vi "KH Control.vi"(8 "error in":errorcluster, 11 "KH7008":refnum<class "Instrument.KH7008.lvclass">) -> (0 "error out":errorcluster, 3 "KH7008.lvclass out":refnum<class "Instrument.KH7008.lvclass">)   [LabVIEW 2019, in "Instrument.KH7008.lvclass"]
uses:
  Instrument.KH7008.lvclass
  typedefs/SetAll-Array.ctl
  typedefs/SetAll-Cluster.ctl
  typedefs/Channel-Enum.ctl
  typedefs/Gain-Enum.ctl
  typedefs/Filter-Enum.ctl
  typedefs/Shunt-Enum.ctl
  typedefs/Coupling-Enum.ctl
  typedefs/Input Configuration-Enum.ctl
  C:/Program Files (x86)/National Instruments/LabVIEW 2019/user.lib/LevyLab/Levylab Instruments/SMOs/Instrument/Instrument.lvclass
  Instrument.KH7008.lvclass/Instrument.KH7008.ctl
  <userlib>/LevyLab/Levylab Instruments/SMOs/Instrument/Instrument.lvclass/Instrument.ctl
  <vilib>/MakerHub/Toolbox/LMH-Toolbox.lvlib
  C:/Program Files (x86)/National Instruments/LabVIEW 2019/vi.lib/JKI/JKI SMO/SMO/SMO.lvclass
  <userlib>/LevyLab/Levylab Instruments/SMOs/Instrument/Instrument.lvclass
panel:
  in  "OK":bool
  in  "Radio Buttons":T1(radio)
  in  "Address":string(combo)="COM3"
  in  "Channel Settings":T2
  # "Measure Current: Current, Shunt Resistor: 50kOhm\nMeasure Voltage: Voltage, Shunt Resistor: Open\nApplying Gate: Current, Shunt Resistor: 50kOhm\n                      Open all the unused gate\n\n1. Create a copy of drivers under C:\\Krohn-Hite 7008\\Drivers if there is none. \n2. In device manager browse the driver for Krohn-Hite \n\nWarning: repeated channels will cause false reading in the lock-in"
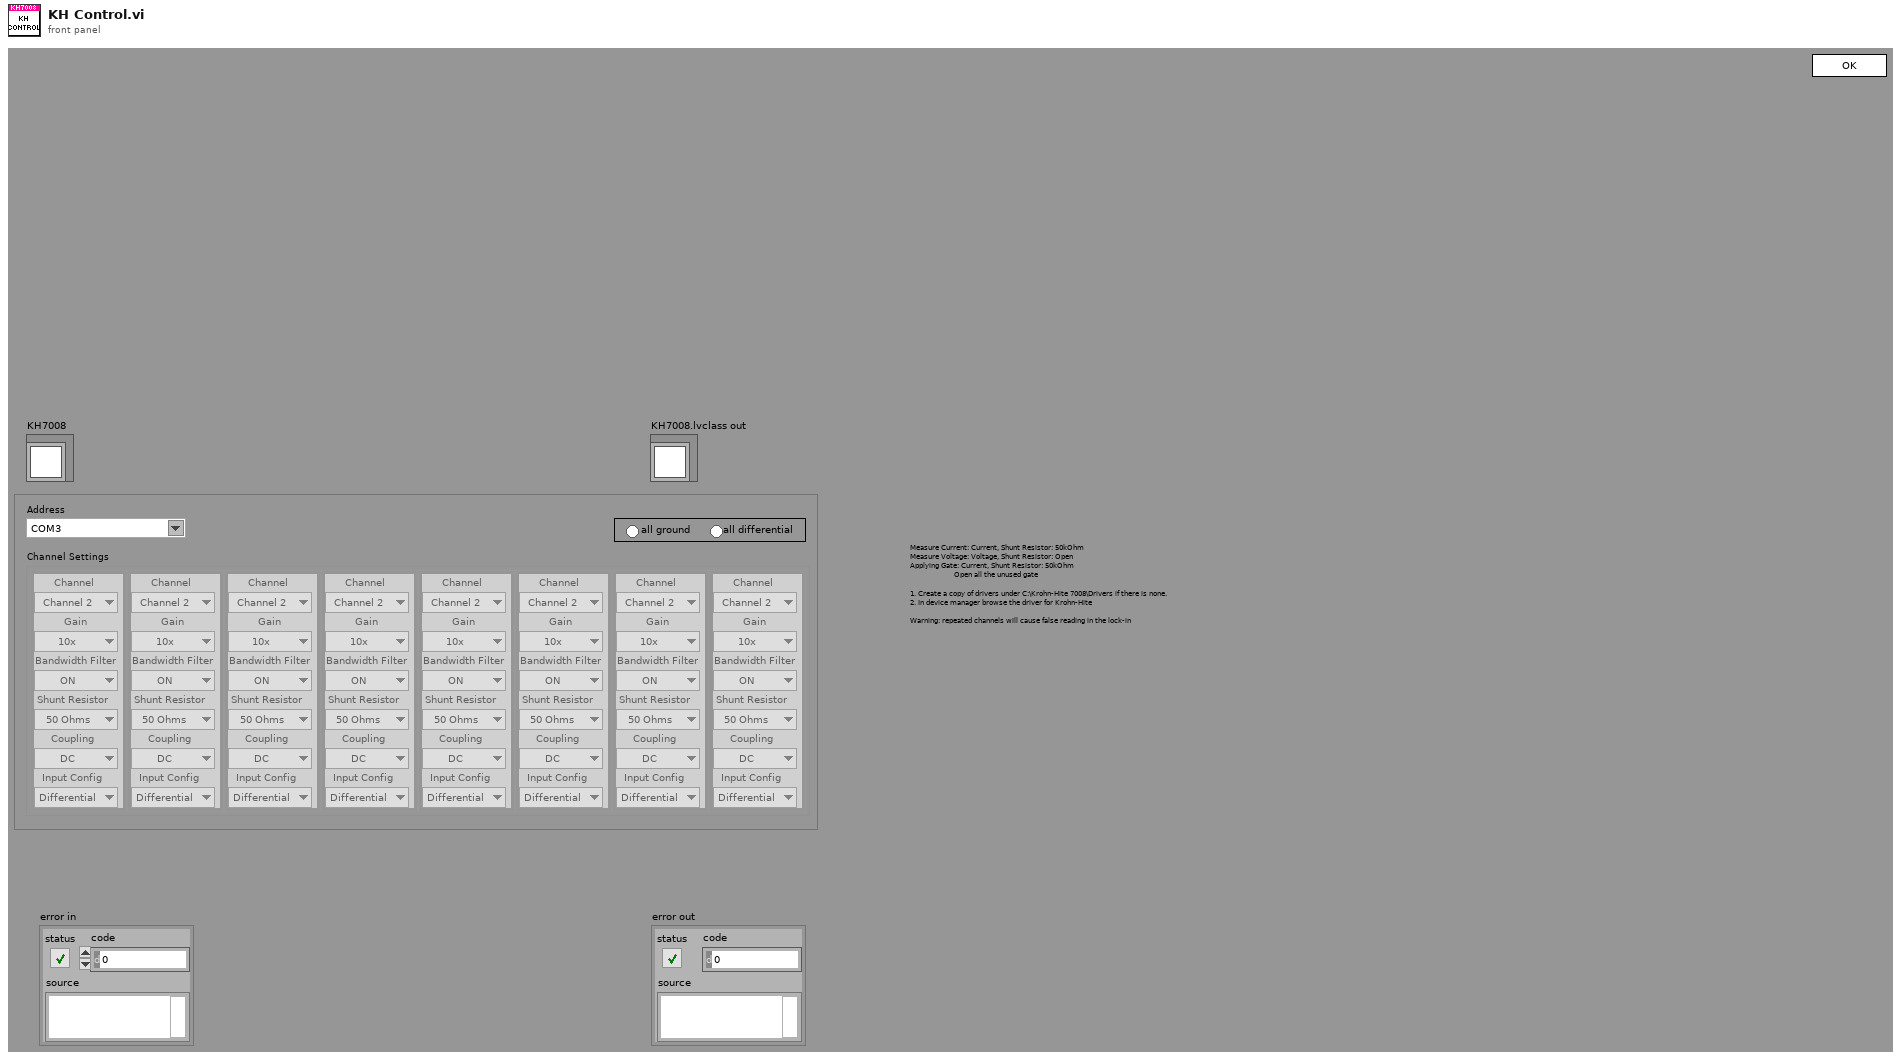
[diagram p1: front panel]
types:
  T1 = enum32{"No Selection", "all ground", "all differential"}
  T2 = typedef "Instrument.KH7008.lvclass/SetAll-Array.ctl" = T3[]
  T3 = typedef "Instrument.KH7008.lvclass/SetAll-Cluster.ctl" = cluster{"Channel":T4, "Gain":T5, "Bandwidth Filter":T6, "Shunt Resistor":T7, "Coupling":T8, "Input Config":T9}
  T4 = typedef "Instrument.KH7008.lvclass/Channel-Enum.ctl" = enum16{"Channel 1", "Channel 2", "Channel 3", "Channel 4", "Channel 5", "Channel 6", "Channel 7", "Channel 8"}
  T5 = typedef "Instrument.KH7008.lvclass/Gain-Enum.ctl" = enum16{"1x", "10x", "100x", "1000x"}
  T6 = typedef "Instrument.KH7008.lvclass/Filter-Enum.ctl" = enum16{"OFF", "ON"}
  T7 = typedef "Instrument.KH7008.lvclass/Shunt-Enum.ctl" = enum16{"Open", "50 Ohms", "500 Ohms", "5k Ohms", "50k Ohms", "10M Ohm"}
  T8 = typedef "Instrument.KH7008.lvclass/Coupling-Enum.ctl" = enum16{"AC", "DC"}
  T9 = typedef "Instrument.KH7008.lvclass/Input Configuration-Enum.ctl" = enum16{"Ground", "SE+ (-gnd)", "SE- (+gnd)", "Differential"}
  T10 = enum32{"Invalid", "Standard", "Closed", "Hidden", "Minimized", "Maximized"}
  T11 = enum32{"invalid app kind", "Development System", "Run Time System", "Student Edition", "Embedded LabVIEW", "Evaluation", "Custom"}
  T12 = cluster{"Core":cluster{"Current VI Reference":refnum<vi>, "Close Panel on Exit?":bool}, "KH7008":refnum<class "Instrument.KH7008.lvclass">, "Address":string, "Channel Setting":T3[]}
  T13 = cluster{"Current VI Reference":refnum<vi>, "Close Panel on Exit?":bool}
  T14 = enum32{"Bad", "Idle", "Run top level", "Running"}
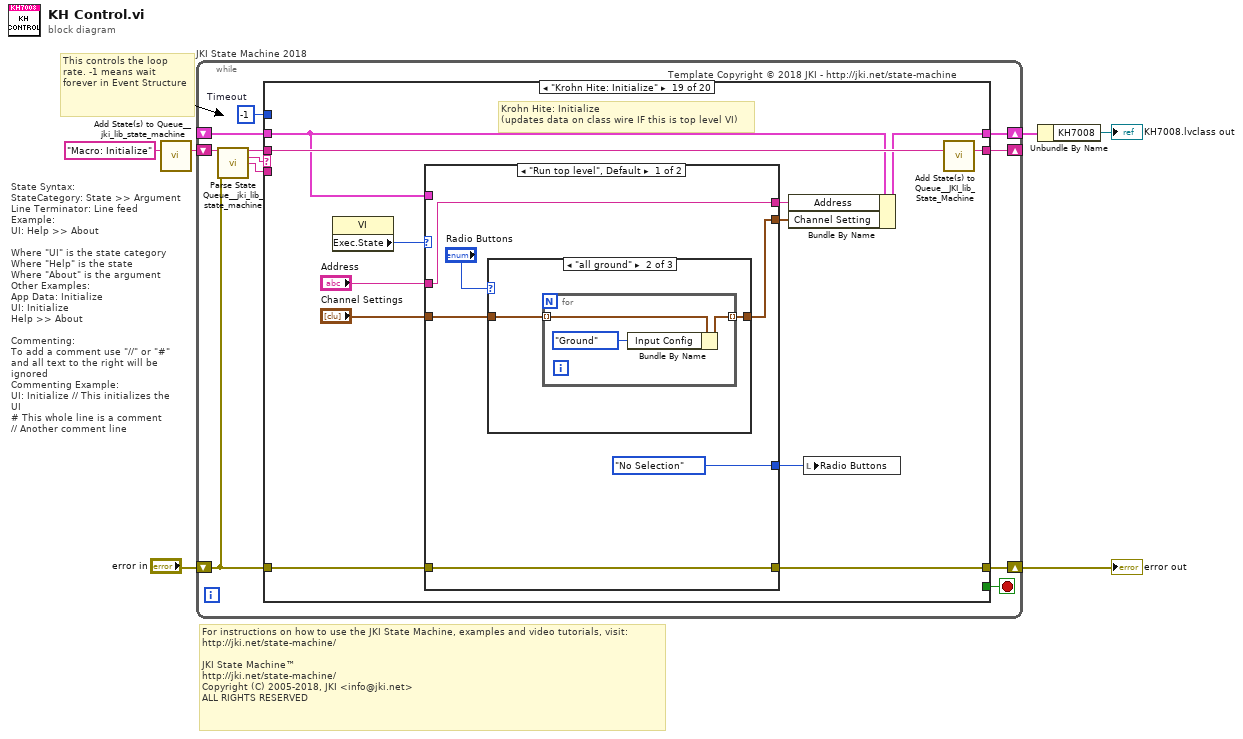
[diagram p0: block diagram]
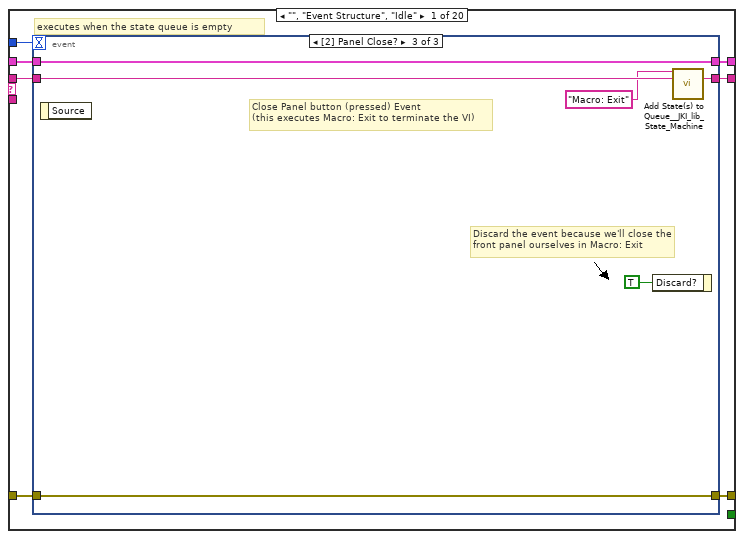
[diagram p2: hidden frame]
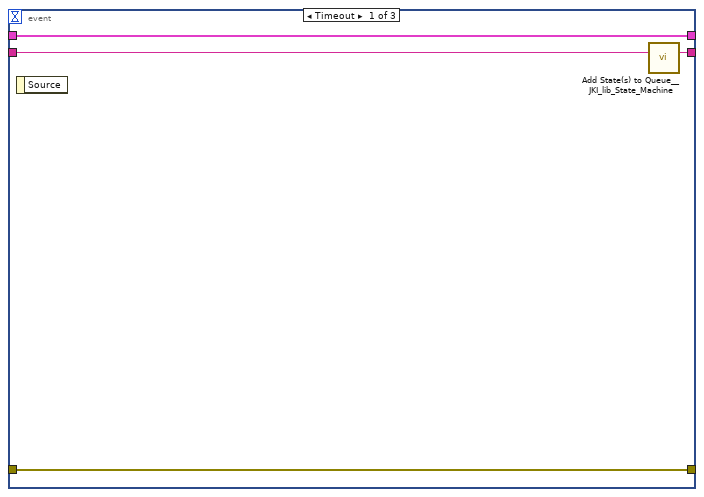
[diagram p3: hidden frame]
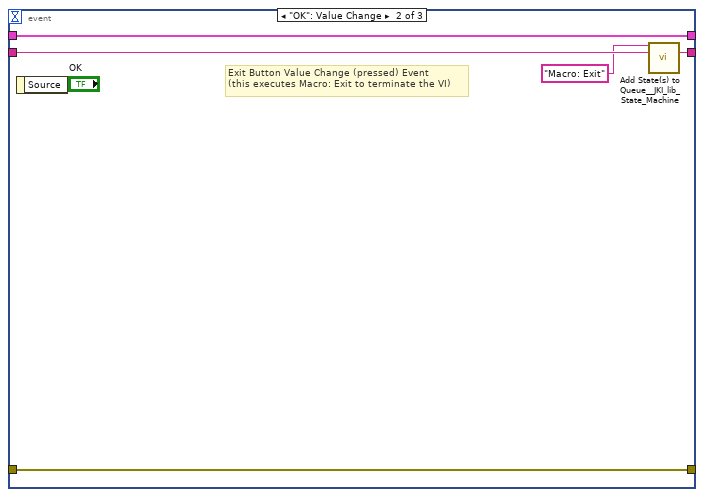
[diagram p4: hidden frame]
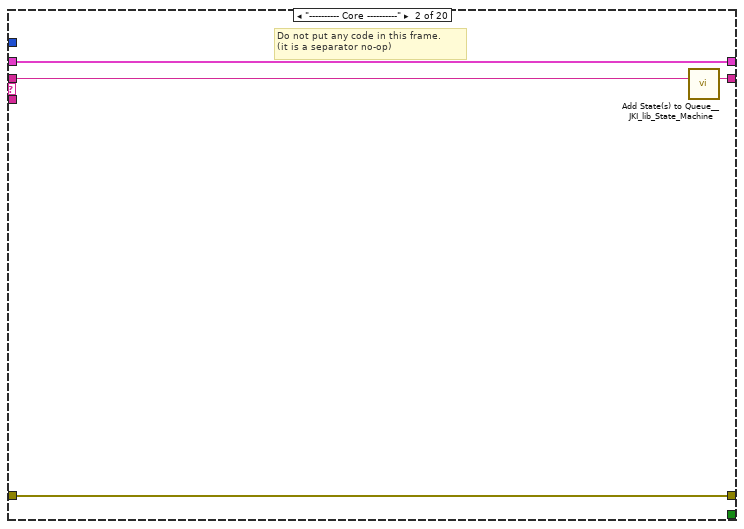
[diagram p5: hidden frame]
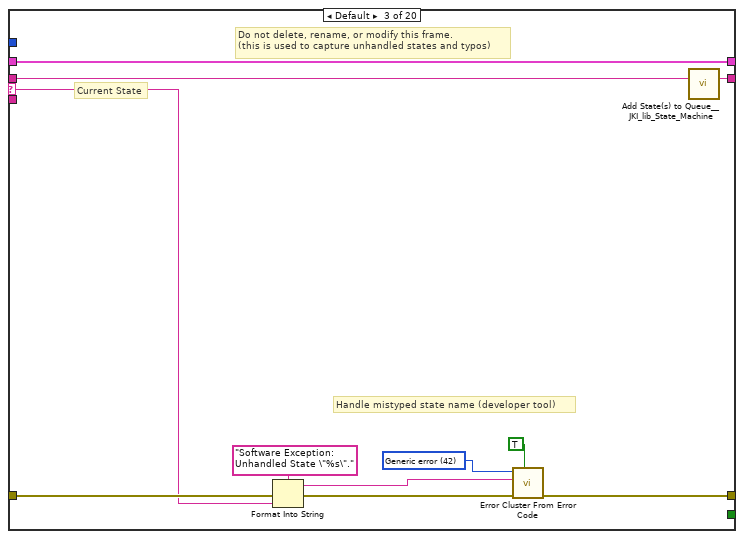
[diagram p6: hidden frame]
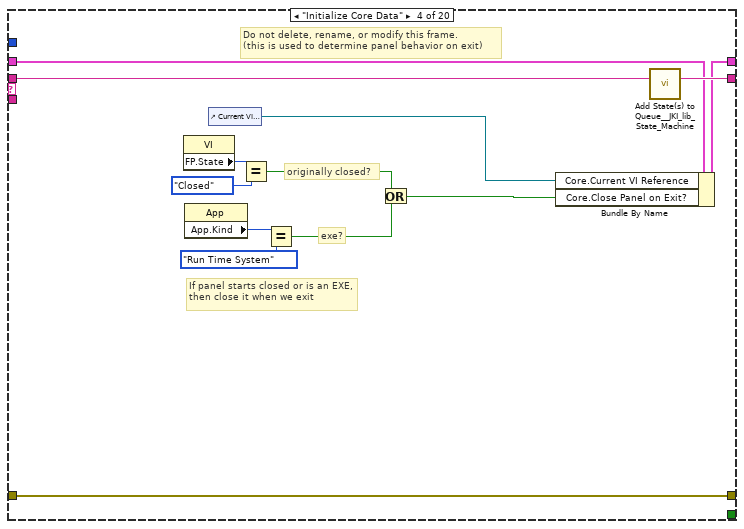
[diagram p7: hidden frame]
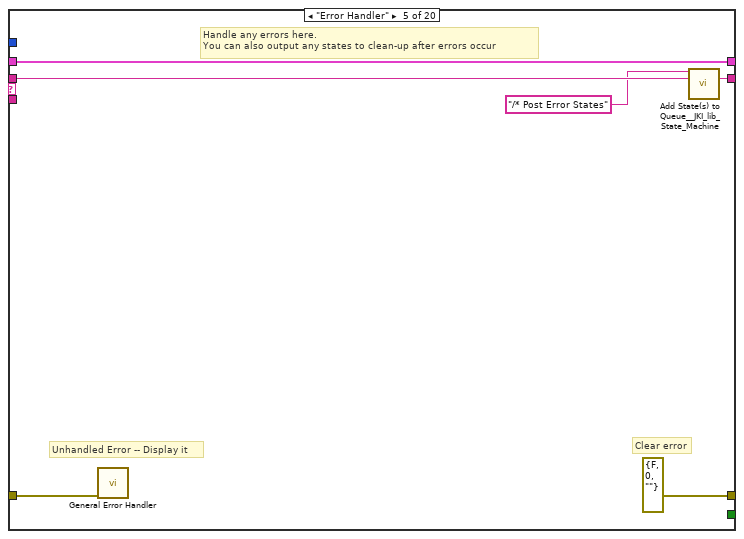
[diagram p8: hidden frame]
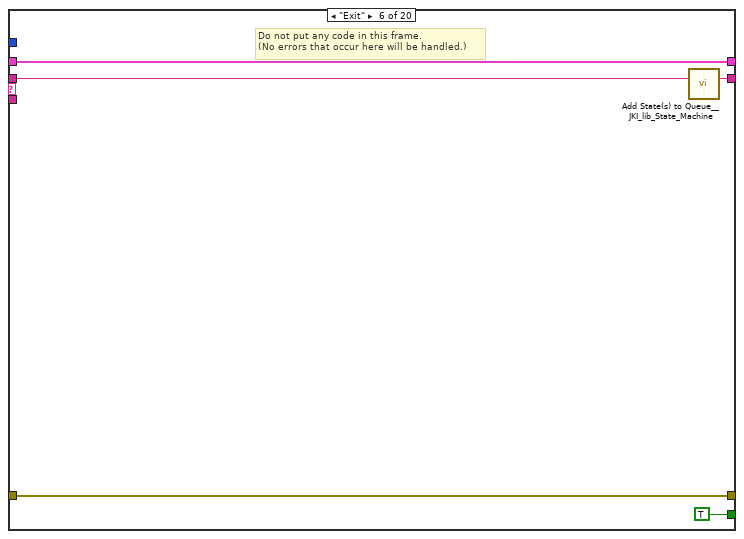
[diagram p9: hidden frame]
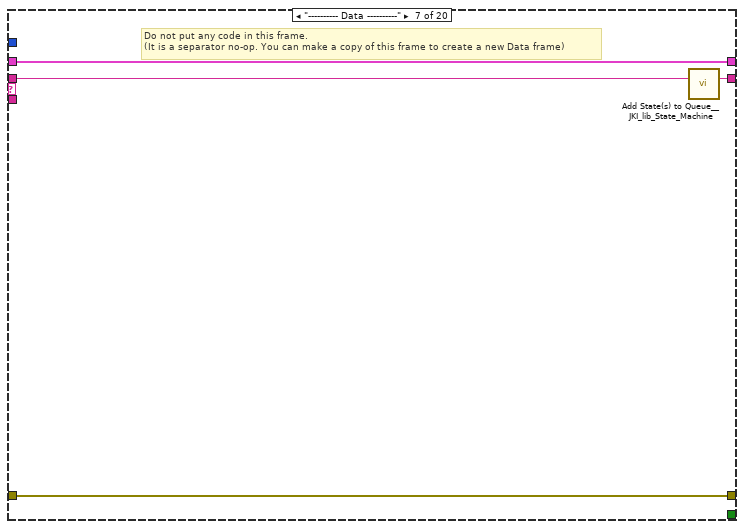
[diagram p10: hidden frame]
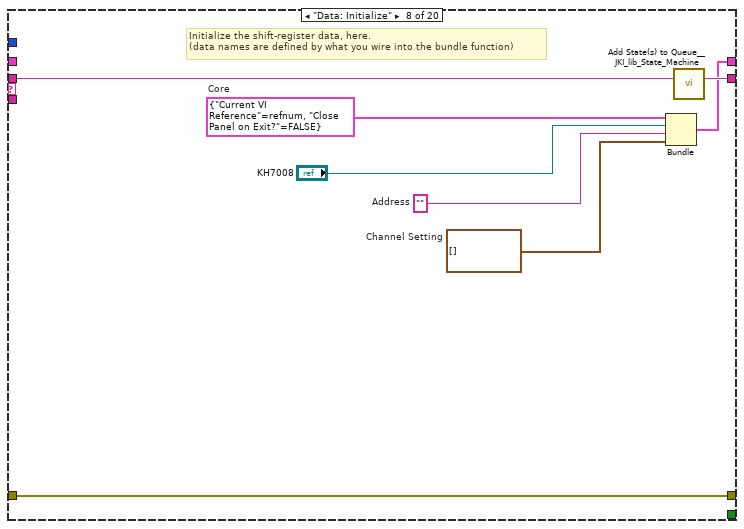
[diagram p11: hidden frame]
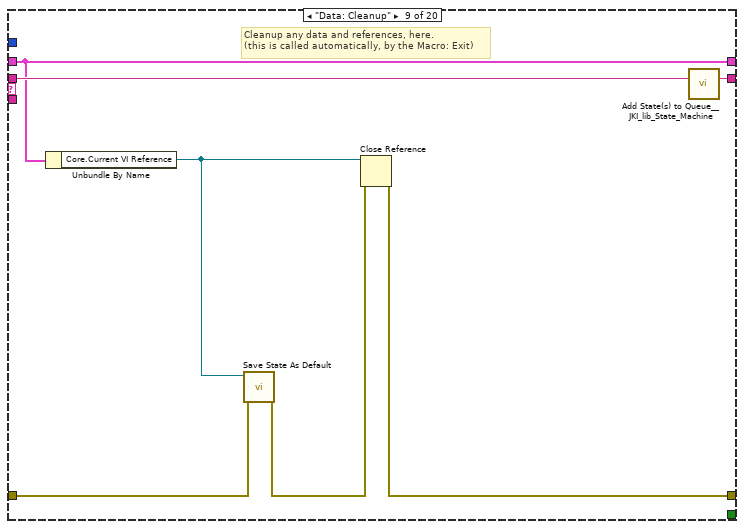
[diagram p12: hidden frame]
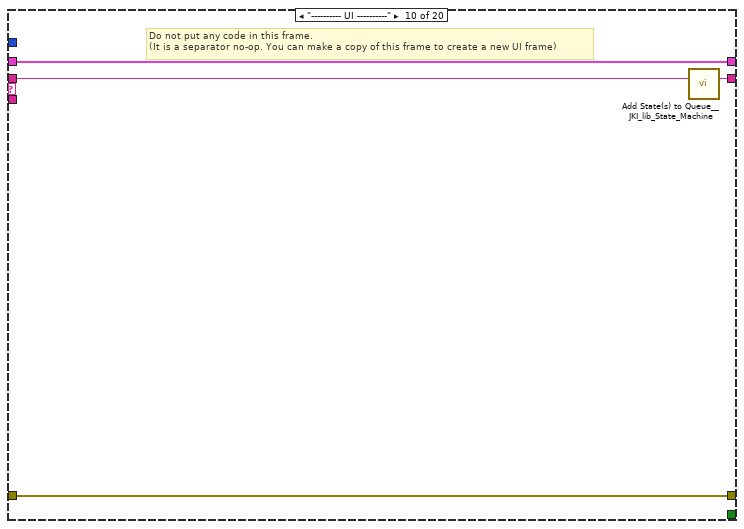
[diagram p13: hidden frame]
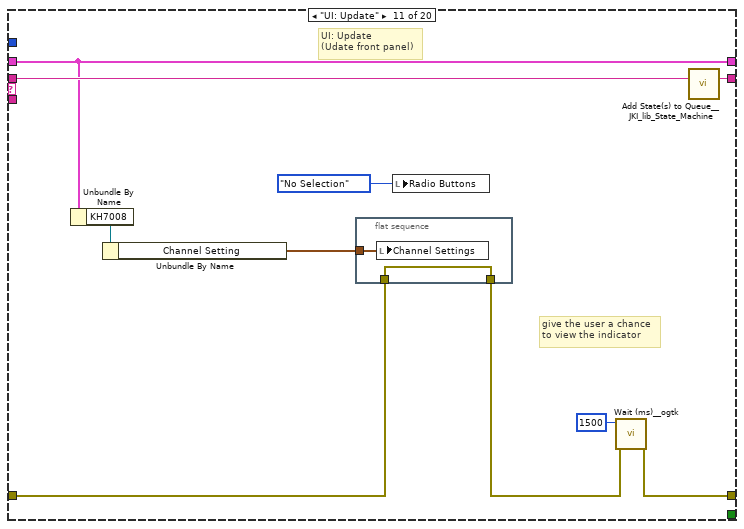
[diagram p14: hidden frame]
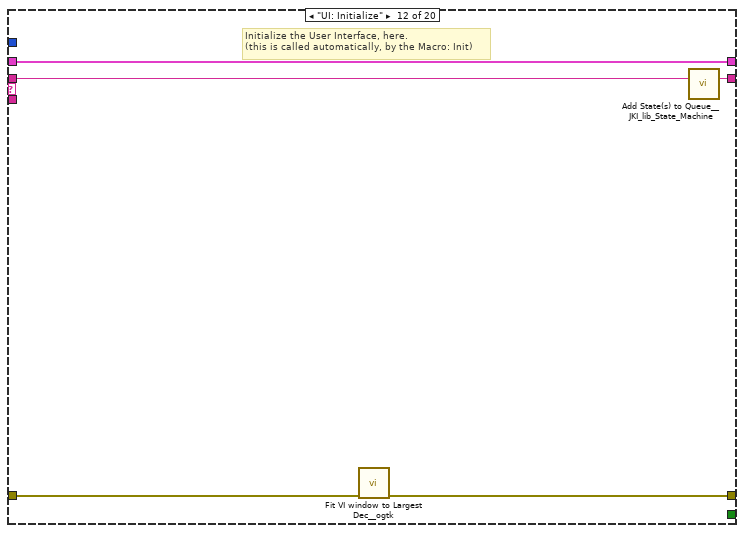
[diagram p15: hidden frame]
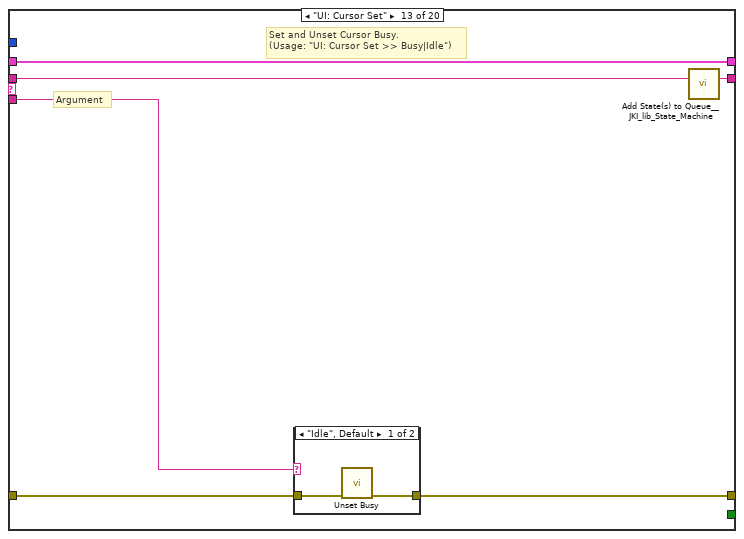
[diagram p16: hidden frame]
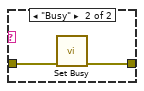
[diagram p17: hidden frame]
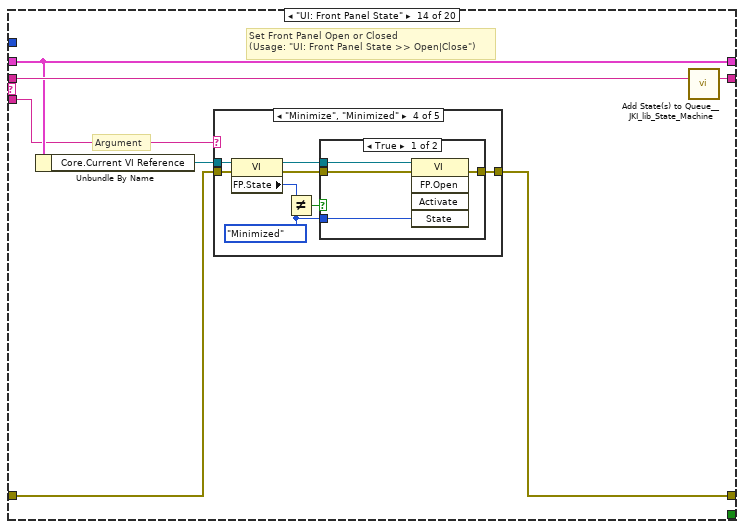
[diagram p18: hidden frame]
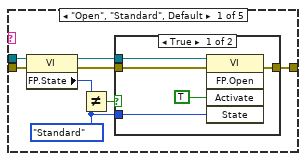
[diagram p19: hidden frame]
diagram:
  # "For instructions on how to use the JKI State Machine, examples and video tutorials, visit:\nhttp://jki.net/state-machine/\n\nJKI State Machine™\nhttp://jki.net/state-machine/\nCopyright (C) 2005-2018, JKI <info@jki.net>\nALL RIGHTS RESERVED"
  # "This controls the loop rate. -1 means wait forever in Event Structure"
  # "State Syntax:\nStateCategory: State >> Argument\nLine Terminator: Line feed\nExample:\nUI: Help >> About\n\nWhere \"UI\" is the state category\nWhere \"Help\" is the state\nWhere \"About\" is the argument\nOther Examples:\nApp Data: Initialize\nUI: Initialize\nHelp >> About\n\nCommenting:\nTo add a comment use \"//\" or \"#\" and all text to the right will be ignored\nCommenting Example:\nUI: Initialize // This initializes the UI\n# This whole line is a comment\n// Another comment line"
  n1 = call <vilib>:"Add State(s) to Queue__jki_lib_state_machine.vi"("State(s) in (\"\")"="Macro: Initialize") -> ("States Out"=w6:string)  [unwired: 14 in]
  n2 = while "JKI State Machine 2018" {
    shift-right: [w7] -> w4
    shift-left: _ -> [w10]
    shift-right: [w13] -> w2
    shift-left: "error in" -> [w8]
    shift-right: [w12] -> _
    shift-left: w6 -> [w14]
    stop <- w11 stop-if-true
    w9 = -1  # Timeout
    # "Template Copyright © 2018 JKI - http://jki.net/state-machine"
    n3 = call <vilib>:"Parse State Queue__jki_lib_state_machine.vi"("State Queue"=w14, "Error In (no error)"=w8) -> ("Remaining States"=w16:string, "Current State"=w17:string, "Arguments"=w15:string)  [unwired: 11 in]
    n4 = case shown="\"Krohn Hite: Initialize\"" w17 {
      selector: w17 -> [_ _ w44 _ _ _ _ _ _ _ _ _ _ _ _ _ _ _ _ _]
      tunnel: w16 -> [w24 w43 w48 w67 w73 w78 w82 w90 w97 w101 w111 w118 w124 w135 w204 w209 w219 w223 w235 w274]
      tunnel: w15 -> [_ _ _ _ _ _ _ _ _ _ _ _ w119 w129 _ _ _ _ _ _]
      tunnel: w10 -> [w22 w40 w46 w60 w70 w76 w79 _ w94 w98 w108 w116 w122 w131 w201 w206 w216 w220 w232 w271]
      tunnel: [w21 w41 w50 w64 errorcluster {"status"=FALSE, "code"=0, "source"=""} ("error out") w75 w80 w86 w95 w99 w105 w114 w120 w132 w202 w207 w217 w221 w227 w262] -> w13
      tunnel: w8 -> [w20 w41 w49 w64 w69 w75 w80 w86 w93 w99 w103 w115 w121 w133 w202 w207 w217 w221 w228 w270]
      tunnel: [w23 w42 w47 w66 w72 w77 w81 w89 w96 w100 w110 w117 w123 w134 w203 w208 w218 w222 w234 w273] -> w12
      tunnel: [_ _ _ _ _ TRUE _ _ _ _ _ _ _ _ _ _ _ _ _ _] -> w11
      tunnel: w9 -> [w18 _ _ _ _ _ _ _ _ _ _ _ _ _ _ _ _ _ _ _]
      tunnel: [w19 w40 w46 w65 w70 w76 w79 w88 w94 w98 w108 w116 w122 w131 w201 w206 w216 w220 w231 w272] -> w7
      frame "", "Event Structure", "Idle" {
        # "executes when the state queue is empty"
        n5 = event shown="[2] Panel Close?" {
          selector: _ -> [_ _ _]
          dyn-events: _ -> [_ _ _]
          timeout: w18 -> [_ _ _]
          tunnel: w24 -> [w28 w33 w39]
          tunnel: [w27 w32 w38] -> w23
          tunnel: w22 -> [w25 w30 w36]
          tunnel: [w26 w31 w37] -> w21
          tunnel: w20 -> [w26 w31 w37]
          tunnel: [w25 w30 w36] -> w19
          event Timeout {
            n6 = event-data() -> ()  [unwired: 1 in, 1 out]
            n7 = call <vilib>:"Add State(s) to Queue__JKI_lib_State_Machine.vi"("State(s) in (\"\")"=w28) -> ("States Out"=w27:string)  [unwired: 14 in]
          }
          event "OK": Value Change {
            # "Exit Button Value Change (pressed) Event\n(this executes Macro: Exit to terminate the VI)"
            n8 = event-data() -> ()  [unwired: 1 in, 1 out]
            n9 = call <vilib>:"Add State(s) to Queue__JKI_lib_State_Machine.vi"("State(s) in Front (\"\")"="Macro: Exit", "State(s) in (\"\")"=w33) -> ("States Out"=w32:string)  [unwired: 13 in]
          }
          event Panel Close? {
            # "Discard the event because we'll close the front panel ourselves in Macro: Exit"
            # "Close Panel button (pressed) Event\n(this executes Macro: Exit to terminate the VI)"
            n10 = event-data() -> ()  [unwired: 1 in, 1 out]
            n11 = event-data("Discard?"=TRUE) -> ()  [unwired: 1 in, 1 out]
            n12 = call <vilib>:"Add State(s) to Queue__JKI_lib_State_Machine.vi"("State(s) in Front (\"\")"="Macro: Exit", "State(s) in (\"\")"=w39) -> ("States Out"=w38:string)  [unwired: 13 in]
          }
        }
      }
      frame "---------- Core ----------" {
        # "Do not put any code in this frame.\n(it is a separator no-op)"
        n13 = call <vilib>:"Add State(s) to Queue__JKI_lib_State_Machine.vi"("State(s) in (\"\")"=w43) -> ("States Out"=w42:string)  [unwired: 14 in]
      }
      frame Default {
        w53 = 42 items=["No error", "Argument error", "Memory is full", "Out of zone", "End of file", "File already open", "Generic file I/O error", "File not found", "File permission error", "Disk is full", "Duplicate path", "Too many files open", "System feature not enabled", "Resource file not found", "Cannot add resource", "Resource not found", "Image not found", "Image memory error", "Pen does not exist", "Config type invalid", "Config token not found", "Config parse error", "Config memory error", "Bad external code format", "Bad external code offset", "External code not present", "Null window", "Destroy window error", "Null menu", "Print aborted", "Bad print record", "Print driver error", "Windows error during printing", "Memory error during printing", "Print dialog error", "Generic print error", "Invalid device refnum", "Device not found", "Device parameter error", "Device unit error", "Cannot open device", "Device call aborted", "Generic error", "Cancelled by user", "Object ID too low", "Object ID too high", "Object not in heap", "Unknown heap", "Unknown object (invalid DefProc)", "Unknown object (DefProc not in table)", "Message out of range", "Invalid (null) method", "Unknown message", "Manager call not supported", "Bad address", "Network operation in progress", "Network operation timed out", "Connection is busy", "Network attribute not supported", "Network error", "Address in use", "System out of memory", "Connection aborted", "Connection refused", "Not connected", "Already connected", "Connection closed", "Initialization error (interapplication manager)", "Bad occurrence", "Wait on unbound occurrence handler", "Occurrence queue overflow", "Datalog type conflict", "Unused", "Unrecognized type (interapplication manager)", "Memory corrupt", "Failed to make temporary DLL", "Old CIN version", "Drag socket not found", "Failed to load drop-object", "Failed to register OLE object", "Failed to release OLE object", "Format specifier type mismatch", "Unknown format specifier", "Too few format specifiers", "Too many format specifiers", "Scan failed", "Newer CIN version", "Error converting to variant", "Runtime menu error", "Password tampered", "Variant attribute not found", "Incompatible variant data type", "Event data is not available", "Event Store is not present", "Occurrence is not found", "Event Queue is not created", "Event info is not available", "Refnum passed is NULL", "Error retrieving Class GUID", "Error retrieving CoClass GUID", "Error retrieving TypeLib GUID.", "Bad built application magic bytes.", "Specific driver is different from the specific driver associated with the Logical Name.", "There is no session opened to the class driver.", "Max Error", "MAX - Error with config objects", "MAX - Error loading configuration", "MAX - Group not supported"]
        # "Current State"
        # "Do not delete, rename, or modify this frame.\n(this is used to capture unhandled states and typos)"
        # "Handle mistyped state name (developer tool)"
        n14 = Format Into String(format string="Software Exception: Unhandled State \"%s\"." ("message"), error in=w49, w44) -> (resulting string=w52:string, error out=w51:errorcluster)  [unwired: 1 in]
        n15 = call <vilib>:"Error Cluster From Error Code.vi"("show call chain? (False)"=TRUE, "error in (no error)"=w51, "error message (\"\")"=w52, "error code (0)"=w53) -> ("error out"=w50:errorcluster)  [unwired: 5 in]
        n16 = call <vilib>:"Add State(s) to Queue__JKI_lib_State_Machine.vi"("State(s) in (\"\")"=w48) -> ("States Out"=w47:string)  [unwired: 14 in]
      }
      frame "Initialize Core Data" {
        # "Do not delete, rename, or modify this frame.\n(this is used to determine panel behavior on exit)"
        # "originally closed?"
        # "exe?"
        # "If panel starts closed or is an EXE, then close it when we exit"
        n17 = property class="VI"() -> ("FP.State"=w57:T10)  [unwired: 2 in, 2 out]
        n18 = property class="App"() -> ("App.Kind"=w63:T11)  [unwired: 2 in, 2 out]
        n19 = control-ref of="Current VI Reference"() -> (w58:refnum<vi>)
        n20 = Equal?(x=w57, y=T10."Closed" ("Front Panel Window:State")) -> (x = y?=w55:bool)
        n21 = Equal?(x=w63, y=T11."Run Time System" ("Application:Kind")) -> (x = y?=w61:bool)
        n22 = Or(x=w55, y=w61) -> (x .or. y?=w59:bool)
        n23 = Bundle By Name(cluster=w60, "Core.Current VI Reference"=w58, "Core.Close Panel on Exit?"=w59) -> (w65:T12)
        n24 = call <vilib>:"Add State(s) to Queue__JKI_lib_State_Machine.vi"("State(s) in (\"\")"=w67) -> ("States Out"=w66:string)  [unwired: 14 in]
      }
      frame "Error Handler" {
        # "Unhandled Error -- Display it"
        # "Handle any errors here.\nYou can also output any states to clean-up after errors occur"
        # "Clear error"
        n25 = call <vilib>:"General Error Handler.vi"("error in (no error)"=w69) -> ()  [unwired: 10 in, 5 out]
        n26 = call <vilib>:"Add State(s) to Queue__JKI_lib_State_Machine.vi"("State(s) in Front (\"\")"="/* Post Error States", "State(s) in (\"\")"=w73) -> ("States Out"=w72:string)  [unwired: 13 in]
      }
      frame "Exit" {
        # "Do not put any code in this frame.\n(No errors that occur here will be handled.)"
        n27 = call <vilib>:"Add State(s) to Queue__JKI_lib_State_Machine.vi"("State(s) in (\"\")"=w78) -> ("States Out"=w77:string)  [unwired: 14 in]
      }
      frame "---------- Data ----------" {
        # "Do not put any code in this frame.\n(It is a separator no-op. You can make a copy of this frame to create a new Data frame)"
        n28 = call <vilib>:"Add State(s) to Queue__JKI_lib_State_Machine.vi"("State(s) in (\"\")"=w82) -> ("States Out"=w81:string)  [unwired: 14 in]
      }
      frame "Data: Initialize" {
        w83 = T3[] []  # Channel Setting
        w84 = ""  # Address
        w87 = T13 {"Current VI Reference"=refnum, "Close Panel on Exit?"=FALSE}  # Core
        # "Initialize the shift-register data, here.\n(data names are defined by what you wire into the bundle function)"
        n29 = Bundle("Core"=w87, "KH7008"="KH7008", "Address"=w84, "Channel Setting"=w83) -> (w88:T12)  [unwired: 1 in]
        n30 = call <vilib>:"Add State(s) to Queue__JKI_lib_State_Machine.vi"("State(s) in (\"\")"=w90) -> ("States Out"=w89:string)  [unwired: 14 in]
      }
      frame "Data: Cleanup" {
        # "Cleanup any data and references, here.\n(this is called automatically, by the Macro: Exit)"
        n31 = Unbundle By Name(w94) -> ("Core.Current VI Reference"=w91:refnum<vi>)
        n32 = call <vilib>:"Save State As Default.vi"("Error In"=w93, "Target VI"=w91) -> ("Error Out"=w92:errorcluster)  [unwired: 8 in, 1 out]
        n33 = Close Reference(reference=w91, error in (no error)=w92) -> (error out=w95:errorcluster)
        n34 = call <vilib>:"Add State(s) to Queue__JKI_lib_State_Machine.vi"("State(s) in (\"\")"=w97) -> ("States Out"=w96:string)  [unwired: 14 in]
      }
      frame "---------- UI ----------" {
        # "Do not put any code in this frame.\n(It is a separator no-op. You can make a copy of this frame to create a new UI frame)"
        n35 = call <vilib>:"Add State(s) to Queue__JKI_lib_State_Machine.vi"("State(s) in (\"\")"=w101) -> ("States Out"=w100:string)  [unwired: 14 in]
      }
      frame "UI: Update" {
        # "give the user a chance\nto view the indicator"
        # "UI: Update\n(Udate front panel)"
        n36 = Unbundle By Name(w108) -> ("KH7008"=w107:refnum<class "Instrument.KH7008.lvclass">)
        n37 = Unbundle By Name(w107) -> ("Channel Setting"=w106:T2)
        n38 = flat-sequence {
          tunnel: w106 -> [w113]
          tunnel: [w112] -> w102
          tunnel: w103 -> [w112]
          frame #0 {
            n39 = local write "Channel Settings"(w113) -> ()
          }
        }
        n40 = local write "Radio Buttons"(T1."No Selection" ("Radio Buttons 2")) -> ()
        n41 = call <userlib>:"Wait (ms)__ogtk.vi"("error in (no error)"=w102, "milliseconds to wait"=u32 1500) -> ("error out"=w105:errorcluster)  [unwired: 8 in, 1 out]
        n42 = call <vilib>:"Add State(s) to Queue__JKI_lib_State_Machine.vi"("State(s) in (\"\")"=w111) -> ("States Out"=w110:string)  [unwired: 14 in]
      }
      frame "UI: Initialize" {
        # "Initialize the User Interface, here.\n(this is called automatically, by the Macro: Init)"
        n43 = call <userlib>:"Fit VI window to Largest Dec__ogtk.vi"("error in (no error)"=w115) -> ("error out"=w114:errorcluster)  [unwired: 5 in, 1 out]
        n44 = call <vilib>:"Add State(s) to Queue__JKI_lib_State_Machine.vi"("State(s) in (\"\")"=w118) -> ("States Out"=w117:string)  [unwired: 14 in]
      }
      frame "UI: Cursor Set" {
        # "Argument"
        # "Set and Unset Cursor Busy.\n(Usage: \"UI: Cursor Set >> Busy|Idle\")"
        n45 = case shown="\"Idle\", Default" w119 {
          tunnel: w121 -> [w126 w128]
          tunnel: [w125 w127] -> w120
          frame "Idle", Default {
            n46 = call <vilib>:"Unset Busy.vi"("error in (no error)"=w126) -> ("error out"=w125:errorcluster)  [unwired: 10 in]
          }
          frame "Busy" {
            n47 = call <vilib>:"Set Busy.vi"("error in (no error)"=w128) -> ("error out"=w127:errorcluster)  [unwired: 9 in, 1 out]
          }
        }
        n48 = call <vilib>:"Add State(s) to Queue__JKI_lib_State_Machine.vi"("State(s) in (\"\")"=w124) -> ("States Out"=w123:string)  [unwired: 14 in]
      }
      frame "UI: Front Panel State" {
        # "Argument"
        # "Set Front Panel Open or Closed\n(Usage: \"UI: Front Panel State >> Open|Close\")"
        n49 = Unbundle By Name(w131) -> ("Core.Current VI Reference"=w130:refnum<vi>)
        n50 = case shown="\"Minimize\", \"Minimized\"" w129 {
          tunnel: w133 -> [w141 w156 w167 w180 w193]
          tunnel: [w143 w157 w169 w182 w195] -> w132
          tunnel: w130 -> [w142 w154 w168 w181 w194]
          frame "Open", "Standard", Default {
            w136 = T10."Standard" ("State")
            n51 = property class="VI"(reference=w142, error in=w141) -> (reference out=w139:refnum<vi>, error out=w140:errorcluster, "FP.State"=w138:T10)
            n52 = Not Equal?(x=w138, y=w136) -> (x != y?=w137:bool)
            n53 = case shown="True" w137 {
              tunnel: [w147 w149] -> w143
              tunnel: w140 -> [w146 w149]
              tunnel: w139 -> [w145 _]
              tunnel: w136 -> [w144 _]
              frame True {
                n54 = invoke class="VI" method="FP.Open"(reference=w145, error in=w146, "Activate"=TRUE, "State"=w144) -> (error out=w147:errorcluster)  [unwired: 1 in, 4 out]
              }
              frame False {
              }
            }
          }
          frame "Close", "Closed" {
            n55 = property class="VI"(reference=w154, error in=w156) -> (reference out=w153:refnum<vi>, error out=w155:errorcluster, "FP.State"=w151:T10)
            n56 = Not Equal?(x=w151, y=T10."Closed" ("Front Panel Window:State")) -> (x != y?=w150:bool)
            n57 = case shown="True" w150 {
              tunnel: [w158 w161] -> w157
              tunnel: w155 -> [w158 w160]
              tunnel: w153 -> [_ w159]
              frame False {
              }
              frame True {
                n58 = invoke class="VI" method="FP.Close"(reference=w159, error in=w160) -> (error out=w161:errorcluster)  [unwired: 1 in, 2 out]
              }
            }
          }
          frame "Hidden", "Hide" {
            w162 = T10."Hidden" ("State")
            n59 = property class="VI"(reference=w168, error in=w167) -> (reference out=w165:refnum<vi>, error out=w166:errorcluster, "FP.State"=w164:T10)
            n60 = Not Equal?(x=w164, y=w162) -> (x != y?=w163:bool)
            n61 = case shown="True" w163 {
              tunnel: [w173 w174] -> w169
              tunnel: w166 -> [w172 w174]
              tunnel: w165 -> [w171 _]
              tunnel: w162 -> [w170 _]
              frame True {
                n62 = invoke class="VI" method="FP.Open"(reference=w171, error in=w172, "State"=w170) -> (error out=w173:errorcluster)  [unwired: 2 in, 4 out]
              }
              frame False {
              }
            }
          }
          frame "Minimize", "Minimized" {
            w175 = T10."Minimized" ("State")
            n63 = property class="VI"(reference=w181, error in=w180) -> (reference out=w178:refnum<vi>, error out=w179:errorcluster, "FP.State"=w177:T10)
            n64 = Not Equal?(x=w177, y=w175) -> (x != y?=w176:bool)
            n65 = case shown="True" w176 {
              tunnel: [w186 w187] -> w182
              tunnel: w179 -> [w185 w187]
              tunnel: w178 -> [w184 _]
              tunnel: w175 -> [w183 _]
              frame True {
                n66 = invoke class="VI" method="FP.Open"(reference=w184, error in=w185, "State"=w183) -> (error out=w186:errorcluster)  [unwired: 2 in, 4 out]
              }
              frame False {
              }
            }
          }
          frame "Maximize", "Maximized" {
            w188 = T10."Maximized" ("State")
            n67 = property class="VI"(reference=w194, error in=w193) -> (reference out=w191:refnum<vi>, error out=w192:errorcluster, "FP.State"=w190:T10)
            n68 = Not Equal?(x=w190, y=w188) -> (x != y?=w189:bool)
            n69 = case shown="True" w189 {
              tunnel: [w199 w200] -> w195
              tunnel: w192 -> [w198 w200]
              tunnel: w191 -> [w197 _]
              tunnel: w188 -> [w196 _]
              frame True {
                n70 = invoke class="VI" method="FP.Open"(reference=w197, error in=w198, "State"=w196) -> (error out=w199:errorcluster)  [unwired: 2 in, 4 out]
              }
              frame False {
              }
            }
          }
        }
        n71 = call <vilib>:"Add State(s) to Queue__JKI_lib_State_Machine.vi"("State(s) in (\"\")"=w135) -> ("States Out"=w134:string)  [unwired: 14 in]
      }
      frame "---------- Macro ----------" {
        # "Do not put any code in this frame.\n(It is a separator no-op. You can make a copy of this frame to create a new Macro frame)"
        n72 = call <vilib>:"Add State(s) to Queue__JKI_lib_State_Machine.vi"("State(s) in (\"\")"=w204) -> ("States Out"=w203:string)  [unwired: 14 in]
      }
      frame "Macro: Initialize" {
        # "Initialization Macro\n(This is called once, when the VI starts)"
        n73 = call <vilib>:"Add State(s) to Queue__JKI_lib_State_Machine.vi"("State(s) in Front (\"\")"="Data: Initialize\nInitialize Core Data\nUI: Initialize\nUI: Front Panel State >> Open\n//\nKrohn Hite: Initialize\nKrohn Hite: Set All\n//\nUI: Update\n//\nMacro: Exit", "State(s) in (\"\")"=w209) -> ("States Out"=w208:string)  [unwired: 13 in]
      }
      frame "Macro: Exit" {
        # "Exit Macro\n(This is called once, when the VI exits)"
        n74 = Unbundle By Name(w216) -> ("Core.Close Panel on Exit?"=w215:bool)
        n75 = Select(t="UI: Front Panel State >> Close", s=w215, f="") -> (s? t:f=w212:string)
        n76 = call <vilib>:"Add State(s) to Queue__JKI_lib_State_Machine.vi"("State(s) in (\"\")"=w212, "State(s) at Back (\"\")"="Data: Cleanup\nExit") -> ("States Out"=w210:string)  [unwired: 13 in]
        n77 = call <vilib>:"Add State(s) to Queue__JKI_lib_State_Machine.vi"("State(s) in Front (\"\")"=w210, "State(s) in (\"\")"=w219) -> ("States Out"=w218:string)  [unwired: 13 in]
      }
      frame "---------- Krohn Hite ----------" {
        # "Template Separator\n(You can make a copy of, or modify, this frame)"
        n78 = call <vilib>:"Add State(s) to Queue__JKI_lib_State_Machine.vi"("State(s) in (\"\")"=w223) -> ("States Out"=w222:string)  [unwired: 14 in]
      }
      frame "Krohn Hite: Initialize" {
        # "Krohn Hite: Initialize\n(updates data on class wire IF this is top level VI)"
        n79 = property class="VI"() -> ("Exec.State"=w233:T14)  [unwired: 2 in, 2 out]
        n80 = case shown="\"Run top level\", Default" w233 {
          tunnel: w232 -> [_ w261]
          tunnel: [w241 w254] -> w230
          tunnel: [w238 w255] -> w229
          tunnel: w228 -> [w240 w258]
          tunnel: [w240 w257] -> w227
          tunnel: "Channel Settings" -> [w239 _]
          tunnel: "Address" -> [w238 _]
          tunnel: [T1."No Selection" ("Radio Buttons") T1."No Selection" ("Radio Buttons")] -> w224
          frame "Run top level", Default {
            n81 = case shown="\"all ground\"" "Radio Buttons" {
              tunnel: [w242 w244 w249] -> w241
              tunnel: w239 -> [w242 w243 w248]
              frame "No Selection", Default {
              }
              frame "all ground" {
                n82 = for {
                  tunnel: w243 -> [w247] mode=indexing
                  tunnel: [w246] -> w244 mode=indexing
                  n83 = Bundle By Name(cluster=w247, "Input Config"=Input_Configuration-Enum."Ground") -> (w246:T3)
                }
              }
              frame "all differential" {
                n84 = for {
                  tunnel: w248 -> [w253] mode=indexing
                  tunnel: [w252] -> w249 mode=indexing
                  n85 = Bundle By Name(cluster=w253, "Input Config"=Input_Configuration-Enum."Differential", "Shunt Resistor"=Shunt-Enum."50k Ohms") -> (w252:T3)
                }
              }
            }
          }
          frame "Running" {
            n86 = Unbundle By Name(w261) -> ("KH7008"=w259:refnum<class "Instrument.KH7008.lvclass">)
            n87 = call <userlib>:"Read Hardware Address.vi"("error in (no error)"=w258, "Instrument in"=w259) -> ("error out"=w257:errorcluster, "Address"=w255:string, "Instrument out"=w256:refnum<class "Instrument.KH7008.lvclass">)  [unwired: 7 in]
            n88 = Unbundle By Name(w256) -> ("Channel Setting"=w254:T2)
          }
        }
        n89 = Bundle By Name(cluster=w232, "Address"=w229, "Channel Setting"=w230) -> (w231:T12)
        n90 = local write "Radio Buttons"(w224) -> ()
        n91 = call <vilib>:"Add State(s) to Queue__JKI_lib_State_Machine.vi"("State(s) in (\"\")"=w235) -> ("States Out"=w234:string)  [unwired: 14 in]
      }
      frame "Krohn Hite: Set All" {
        # "Your code here.\n(You can make a copy of, or modify, this frame)"
        n92 = Unbundle By Name(w271) -> ("KH7008"=w267:refnum<class "Instrument.KH7008.lvclass">, "Address"=w268:string, "Channel Setting"=w266:T3[])
        n93 = call "KH7008 Set All Channels.vi"("error in (no error)"=w270, "Channel Params []"=w266, "VISA Refnum in"=w268) -> ("error out"=w263:errorcluster, "Ch Params [] out"=w264:T3[])  [unwired: 6 in, 1 out]
        n94 = call "KH7008 Get All Channel Gains.vi"("error in (no error)"=w263, "Channel Params []"=w264) -> ("error out"=w262:errorcluster, "Gains []"=w265:dbl[])  [unwired: 8 in]
        n95 = Bundle By Name(cluster=w267, "Channel Setting"=w264, "Gain"=w265) -> (w269:refnum<class "Instrument.KH7008.lvclass">)
        n96 = Bundle By Name(cluster=w271, "KH7008"=w269) -> (w272:T12)
        n97 = call <vilib>:"Add State(s) to Queue__JKI_lib_State_Machine.vi"("State(s) in (\"\")"=w274) -> ("States Out"=w273:string)  [unwired: 14 in]
      }
    }
  }
  "error out" <- w2
  n98 = Unbundle By Name(w4) -> ("KH7008"=→"KH7008.lvclass out":refnum<class "Instrument.KH7008.lvclass">)
